vi "ParseVisionData.vi"(8 "error in (no error)":errorcluster, 11 "JSON String":string) -> (1 "Boolean Data":T1, 3 "Distance and Angle":cluster{"Distance":dbl, "Angle":dbl})   [LabVIEW 2015]
uses:
  <vilib>/Rock Robotics/Network Tables/NT Write String.vi
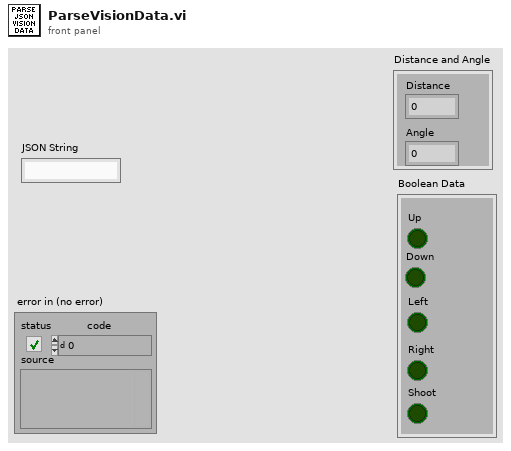
[diagram p1: front panel]
types:
  T1 = cluster{"Up":bool, "Down":bool, "Left":bool, "Right":bool, "Shoot":bool}
  T2 = cluster{"Distance":string, "Angle":string, "Up":string, "Down":string, "Left":string, "Right":string, "Shoot":string}
  T3 = cluster{"Boolean":bool, "Boolean":bool, "Boolean":bool, "Boolean":bool, "Boolean":bool}
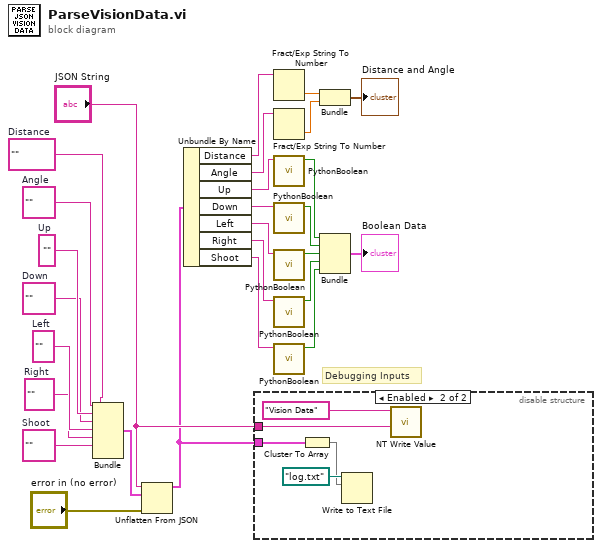
[diagram p0: block diagram]
diagram:
  w3 = ""  # Shoot
  w4 = ""  # Right
  w7 = ""  # Up
  w6 = ""  # Down
  w5 = ""  # Left
  w8 = ""  # Angle
  w9 = ""  # Distance
  # "Debugging Inputs"
  n1 = Bundle("Distance"=w9, "Angle"=w8, "Up"=w7, "Down"=w6, "Left"=w5, "Right"=w4, "Shoot"=w3) -> (w2:T2)  [unwired: 1 in]
  n2 = Unflatten From JSON(JSON string="JSON String", type and defaults=w2, error in (no error)="error in (no error)") -> (value=w1:T2)  [unwired: 4 in, 1 out]
  n3 = Unbundle By Name(w1) -> ("Distance"=w27:string, "Angle"=w26:string, "Up"=w23:string, "Down"=w21:string, "Left"=w20:string, "Right"=w19:string, "Shoot"=w18:string)
  n4 = disable-structure shown="Enabled" {
    disable-tunnel: w1 -> [_ w32]
    disable-tunnel: "JSON String" -> [_ w28]
    frame Disabled {
    }
    frame Enabled {
      n5 = Cluster To Array(cluster=w32) -> (array=w30:string[])
      n6 = Write to Text File(file (use dialog)=path "log.txt", text=w30) -> ()  [unwired: 2 in, 3 out]
      n7 = call-poly <vilib>:"NT Write Value.vi"("String"=w28, "Name"="Vision Data") -> ()  [unwired: 9 in, 1 out]
    }
  }
  n8 = Fract/Exp String To Number(string=w27) -> (number=w25:dbl)  [unwired: 3 in, 1 out]
  n9 = Fract/Exp String To Number(string=w26) -> (number=w24:dbl)  [unwired: 3 in, 1 out]
  n10 = call "PythonBoolean.vi"("Python Boolean as String"=w23) -> ("Boolean"=w22:bool)  [unwired: 10 in]
  n11 = call "PythonBoolean.vi"("Python Boolean as String"=w21) -> ("Boolean"=w17:bool)  [unwired: 10 in]
  n12 = call "PythonBoolean.vi"("Python Boolean as String"=w20) -> ("Boolean"=w16:bool)  [unwired: 10 in]
  n13 = call "PythonBoolean.vi"("Python Boolean as String"=w19) -> ("Boolean"=w15:bool)  [unwired: 10 in]
  n14 = call "PythonBoolean.vi"("Python Boolean as String"=w18) -> ("Boolean"=w14:bool)  [unwired: 10 in]
  n15 = Bundle(w25, w24) -> (→"Distance and Angle":cluster{dbl, dbl})  [unwired: 1 in]
  n16 = Bundle("Boolean"=w22, "Boolean"=w17, "Boolean"=w16, "Boolean"=w15, "Boolean"=w14) -> (→"Boolean Data":T3)  [unwired: 1 in]
